vi "Initialize.vi"(8 "Error In":errorcluster) -> (0 "Error Out":errorcluster)   [LabVIEW 2012]
uses:
  <vilib>/robotics/Simulator/NI_Robotics_Simulator.lvlib
panel:
  in  "Sim ID":T1(array[cluster])=[{"Robot"="Husky Demo_R0", "Sensors"=["GPS_S0", "LIDAR_S0", "IMU_S0", "Compass_S0", "Camera_S0"], "Joints"=["Front Right Joint", "Rear Right Joint", "Rear Left Joint", "Front Left Joint"], "Actuators"=["Front Right Motor", "Rear Right Motor", "Rear Left Motor", "Front Left Motor"], "Robot Components"=["ID4", "Front Left Wheel", "Rear Left Wheel", "Front Right Wheel", "Rear Right Wheel"]}]
  in  "manifest filename":string="Husky Demo\\Husky Demo Simulation.xml"
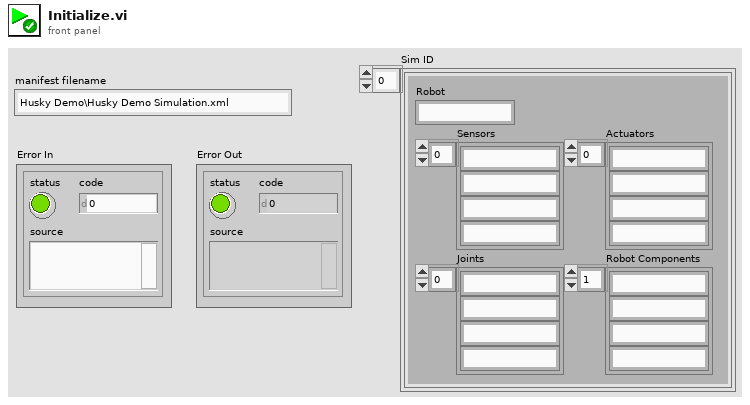
[diagram p1: front panel]
types:
  T1 = cluster{"Robot":string, "Sensors":string[], "Joints":string[], "Actuators":string[], "Robot Components":string[]}[]
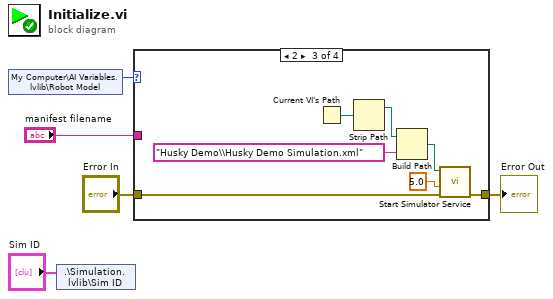
[diagram p0: block diagram]
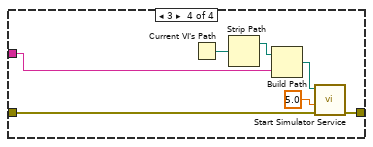
[diagram p4: hidden frame]
diagram:
  n1 = shared-variable "My Computer\\AI Variables.lvlib\\Robot Model"() -> (w5:u16)  [unwired: 1 in, 1 out]
  n2 = shared-variable ".\\Simulation.lvlib\\Sim ID"("Sim ID") -> ()  [unwired: 1 in, 1 out]
  n3 = case shown="2" w5 {
    tunnel: [w6 w7 w9 w16] -> w4
    tunnel: "Error In" -> [w6 w7 w10 w17]
    tunnel: "manifest filename" -> [_ _ _ w15]
    frame 0, Default {
    }
    frame 1 {
    }
    frame 2 {
      n4 = Current VI's Path() -> (path=w12:path)
      n5 = Strip Path(path=w12) -> (stripped path=w13:path)  [unwired: 1 out]
      n6 = Build Path(base path=w13, name or relative path="Husky Demo\\Husky Demo Simulation.xml" ("manifest filename 2")) -> (appended path=w14:path)
      n7 = call <vilib>:"Start Simulator Service.vi"("error in (no error)"=w10, "step size (ms)"=5.0 ("stepsize(ms)"), "manifest file"=w14) -> ("error out"=w9:errorcluster)  [unwired: 8 in]
    }
    frame 3 {
      n8 = Current VI's Path() -> (path=w19:path)
      n9 = Strip Path(path=w19) -> (stripped path=w20:path)  [unwired: 1 out]
      n10 = Build Path(base path=w20, name or relative path=w15) -> (appended path=w21:path)
      n11 = call <vilib>:"Start Simulator Service.vi"("error in (no error)"=w17, "step size (ms)"=5.0 ("stepsize(ms)"), "manifest file"=w21) -> ("error out"=w16:errorcluster)  [unwired: 8 in]
    }
  }
  "Error Out" <- w4
